vi "Set 1D DBL Read Q on Variant.vi"(8 "error in (no error)":errorcluster, 10 "1D DBL Read Q":T1, 11 "Variant in":variant) -> (0 "error out":errorcluster, 2 "replaced":bool, 3 "Variant out":variant)   [LabVIEW 2020, in "Internal Comm Classes.lvlib" / "WPL Comm (1D DBL).lvclass"]
uses:
  WPL Comm (1D DBL).lvclass
  Waveform 1d dbl read queue.ctl
  Waveform 1d dbl read cluster.ctl
  Waveform properties.ctl
  Custom Device API/Waveform Data Reference.ctl
  NI_VS Custom Device Waveform API.lvlib
  Custom Device API/Custom Device API.lvlib
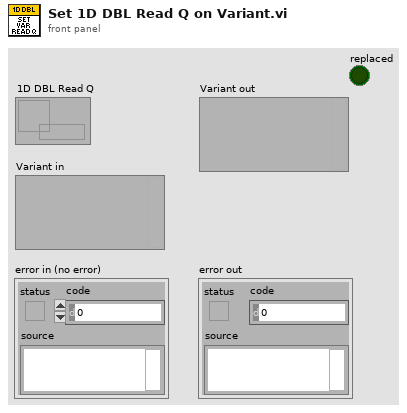
[diagram p1: front panel]
types:
  T1 = typedef "Internal Comm Classes.lvlib/WPL Comm (1D DBL).lvclass/Waveform 1d dbl read queue.ctl" = refnum<queue>
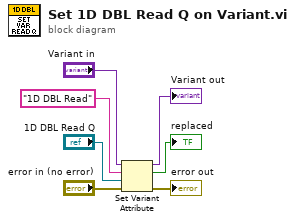
[diagram p0: block diagram]
diagram:
  n1 = Set Variant Attribute(Variant="Variant in", name="1D DBL Read", value="1D DBL Read Q", error in="error in (no error)") -> (Variant out=→"Variant out":variant, replaced=→"replaced":bool, error out=→"error out":errorcluster)
